vi "Get VI Ref.vi"(8 "error in":errorcluster, 11 "vi id":string) -> (0 "error out":errorcluster, 3 "vi ref":refnum<vi>)   [LabVIEW 2026, in "G-AI Core.lvlib"]
uses:
  G-AI Core.lvlib
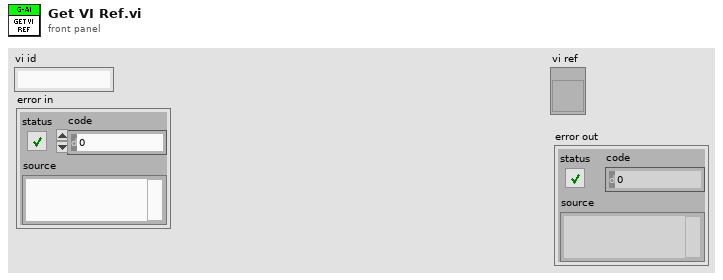
[diagram p1: front panel]
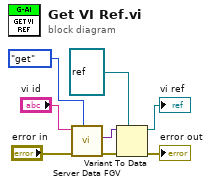
[diagram p0: block diagram]
diagram:
  n1 = call "Server Data FGV.vi"("mode"=enum16{"get", "set", "reset"}."get", "error in"="error in", "name (empty=auto)"="vi id") -> ("error out"=w5:errorcluster, "data out"=w4:variant)  [unwired: 5 in, 2 out]
  n2 = Variant To Data(error in=w5, type=refnum<vi> refnum ("vi reference"), Variant=w4) -> (data=→"vi ref":refnum<vi>, error out=→"error out":errorcluster)
